vi "close.vi"(8 "error IO":errorcluster) -> (0 "error":errorcluster)   [LabVIEW 2013, in "PicoMotor.lvclass"]
uses:
  PicoMotor.lvclass
  PicoMotor.lvclass/PicoMotor.ctl
  Globals.vi
panel:
  out "PicoMotor":refnum<class "PicoMotor.lvclass">
  in  "PicoMotor (in)":refnum<class "PicoMotor.lvclass">
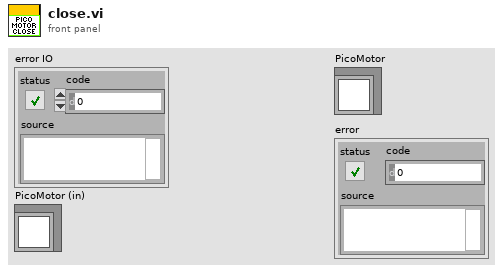
[diagram p1: front panel]
types:
  T1 = typedef "Experiment.lvclass/states.ctl" = enum16{"run", "pause", "shutdown gracefully", "halt immediately", "waiting for connection", "waiting for command"}
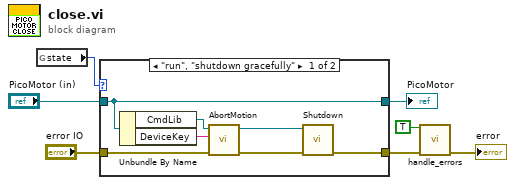
[diagram p0: block diagram]
diagram:
  n1 = global read "Globals.vi" "state"() -> (w5:T1)
  n2 = case shown="\"run\", \"shutdown gracefully\"" w5 {
    tunnel: [w12 w16] -> w7
    tunnel: "error IO" -> [w9 w16]
    tunnel: "PicoMotor (in)" -> [w8 w15]
    tunnel: [w8 w15] -> w2
    frame "run", "shutdown gracefully" {
      n3 = Unbundle By Name(w8) -> ("CmdLib"=w11:refnum<k24>, "DeviceKey"=w10:string)
      n4 = call "AbortMotion.vi"("error in (no error)"=w9, "DeviceKey In"=w10, "CmdLib In"=w11) -> ("error out"=w14:errorcluster, "CmdLib Out"=w13:refnum<k24>)  [unwired: 2 in, 1 out]
      n5 = call "Shutdown.vi"("error in (no error)"=w14, "CmdLib In"=w13) -> ("error out"=w12:errorcluster)  [unwired: 4 in, 1 out]
    }
    frame Default {
    }
  }
  "PicoMotor" <- w2
  n6 = call "handle_errors.vi"("Exit Operation"=TRUE, "error in (no error)"=w7) -> ("error out"=→"error":errorcluster)  [unwired: 13 in]
